vi "UT_009_Get TOML data.vi"   [LabVIEW 2017]
uses:
  092c8865-a0f3-441c-b4b4-216df50b1920.vi
  78aca855-5324-48c4-8215-c8667f1e6632.vi
  lib/TOML to LabVIEW.vi
  <vilib>/addons/_JKI Toolkits/Caraya/classes/Assert/Assert Equal Value_Variant.vi
  <vilib>/addons/_JKI Toolkits/Caraya/classes/Test/Test.lvclass
  <vilib>/addons/_JKI Toolkits/Caraya/classes/Assert/Assert.lvclass
  lib/TOML.lvlib
types:
  T1 = cluster{"cluster":cluster{"string":string, "bool":bool, "path":path, "DBL":dbl}, "1d-array-cluster":cluster{"string":string, "int":i32, "SGL":sgl}[]}
  T2 = typedef "TOML.lvlib/TOML Value.ctl" = cluster{"type":enum16{"Table", "Array", "String", "Integer", "Float", "Boolean", "Offset Date-Time", "Local Date-Time", "Local Date", "Local Time", "Path"}, "value":variant}
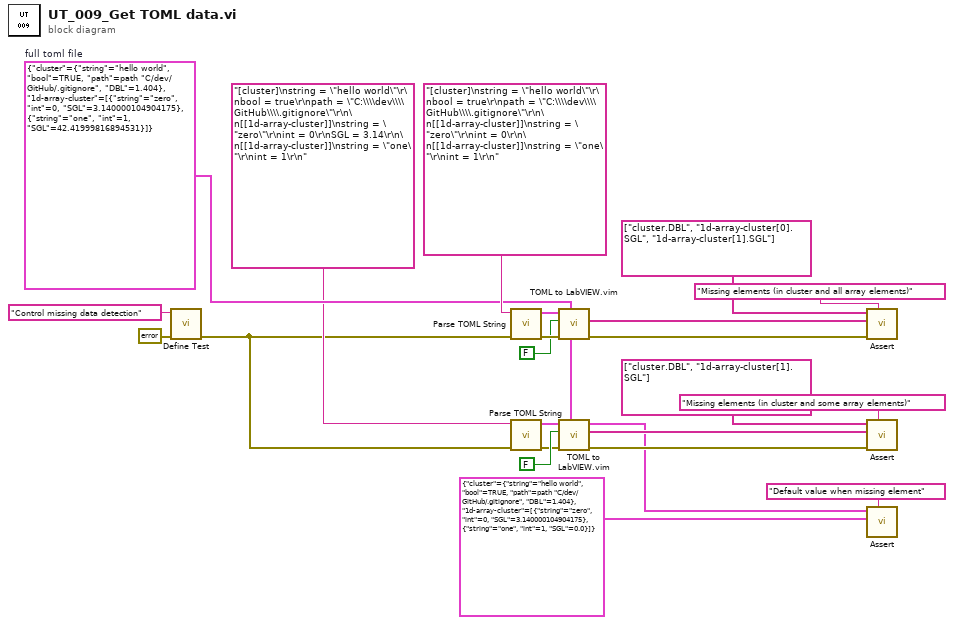
[diagram p0: block diagram]
diagram:
  w10 = T1 {"cluster"={"string"="hello world", "bool"=TRUE, "path"=path "C:/dev/GitHub/.gitignore", "DBL"=1.404}, "1d-array-cluster"=[{"string"="zero", "int"=0, "SGL"=3.14}, {"string"="one", "int"=1, "SGL"=42.42}]}  # full toml file
  n1 = call <vilib>:"Define Test.vi"("error in (no error)"=errorcluster {"status"=FALSE, "code"=0, "source"=""}, "Label (VI Title)"="Control missing data detection") -> ("error out"=w4:errorcluster)  [unwired: 9 in]
  n2 = call "Parse TOML String.vi"("error in (no error)"=w4, "String"="[cluster]\nstring = \"hello world\"\r\nbool = true\r\npath = \"C:\\\\dev\\\\GitHub\\\\.gitignore\"\r\n\n[[1d-array-cluster]]\nstring = \"zero\"\r\nint = 0\r\n\n[[1d-array-cluster]]\nstring = \"one\"\r\nint = 1\r\n" ("x")) -> ("error out"=w20:errorcluster, "Value"=w19:T2)  [unwired: 8 in]
  n3 = call "Parse TOML String.vi"("error in (no error)"=w4, "String"="[cluster]\nstring = \"hello world\"\r\nbool = true\r\npath = \"C:\\\\dev\\\\GitHub\\\\.gitignore\"\r\n\n[[1d-array-cluster]]\nstring = \"zero\"\r\nint = 0\r\nSGL = 3.14\r\n\n[[1d-array-cluster]]\nstring = \"one\"\r\nint = 1\r\n" ("x")) -> ("error out"=w12:errorcluster, "Value"=w13:T2)  [unwired: 8 in]
  n4 = call "TOML to LabVIEW.vim"("datatype"=w10, "error in (no error)"=w20, "Error if missing element"=FALSE, "Value"=w19) -> ("error out"=w17:errorcluster, "Missing elements"=w16:string[])  [unwired: 5 in, 1 out]
  n5 = call "TOML to LabVIEW.vim"("datatype"=w10, "error in (no error)"=w12, "Error if missing element"=FALSE, "Value"=w13) -> ("error out"=w6:errorcluster, "Missing elements"=w8:string[], "LV Data"=w3:T1)  [unwired: 5 in]
  n6 = call-poly <vilib>:"Assert.vi"("Label"="Missing elements (in cluster and all array elements)" ("Label (VI Title)"), "error in (no error)"=w17, "Y"=w16, "X"=string[] ["cluster.DBL", "1d-array-cluster[0].SGL", "1d-array-cluster[1].SGL"] ("Missing elements")) -> ()  [unwired: 7 in, 1 out]
  n7 = call-poly <vilib>:"Assert.vi"("Label"="Missing elements (in cluster and some array elements)" ("Label (VI Title)"), "error in (no error)"=w6, "Y"=w8, "X"=string[] ["cluster.DBL", "1d-array-cluster[1].SGL"] ("Missing elements")) -> ()  [unwired: 7 in, 1 out]
  n8 = call-poly <vilib>:"Assert.vi"("Label"="Default value when missing element" ("Label (VI Title)"), "Y"=T1 {"cluster"={"string"="hello world", "bool"=TRUE, "path"=path "C:/dev/GitHub/.gitignore", "DBL"=1.404}, "1d-array-cluster"=[{"string"="zero", "int"=0, "SGL"=3.14}, {"string"="one", "int"=1, "SGL"=0.0}]} ("LV Data"), "X"=w3) -> ()  [unwired: 8 in, 1 out]
